vi "shag_start — 6.vi"() -> ()   [LabVIEW 2016]
uses:
  <vilib>/Instr/_visa.llb/VISA Configure Serial Port (Instr).vi
panel:
  out "file":i32
  out "положение в мин 1":i32
  in  "all":T1(tab)
  out "положение шд":i32(knob) scale=-10.0..190.0
  out "текущее положение":string
  out "положение в минутах 1":string
  in  "Минуты":i32 min=-600 max=11400
  in  "Stop двигатель":bool
  in  "Вращение по градусам +":bool
  in  "Вращение по градусам -":bool
  in  "Вернуться в нулевое положение":bool
  in  "Задать текущее положение нулевым":bool
  in  "Установка минут":bool
  in  "Блокировать зеркало №1":bool
  in  "stop":bool
  in  "Выберете COM порт":refnum<visa-resource-name>="COM1"
  in  "Скорость обмена данными":u32(ring)=19200 items=["9600"=9600, "19200"=19200, "38400"=38400, "57600"=57600]
  in  "Число бит на символ":u16=8 min=5 max=8 step=1
  in  "Контроль чётности":enum16{"None", "Odd", "Even", "Mark", "Space"}(ring)
  in  "Стоповый бит":u16(ring)=10 items=["1.0"=10, "1.5"=15, "2.0"=20]
  in  "Контроль переполнения":u16(ring) items=["None"=0, "XON/XOFF"=1, "RTS/CTS"=2, "DTR/DSR"=4]
  # "1 - адресс 1 двигателя\n2 - адресс 2 двигателя\n$0MV\\01+   - запуск всех двигателей в положительном направлении \n$0MS\\00   - остановка всех двигателей\n$0MJ\\04+\\00\\00\\01   - 1 шаг всех двигателей\n$0SS\\01\\10   - скорость 10 для всех двигателей"
  # "Зеркало №1"
  # "Положение:"
  # "Ренгеновская трубка №2:"
  # "Положение ренгеновской трубк:"
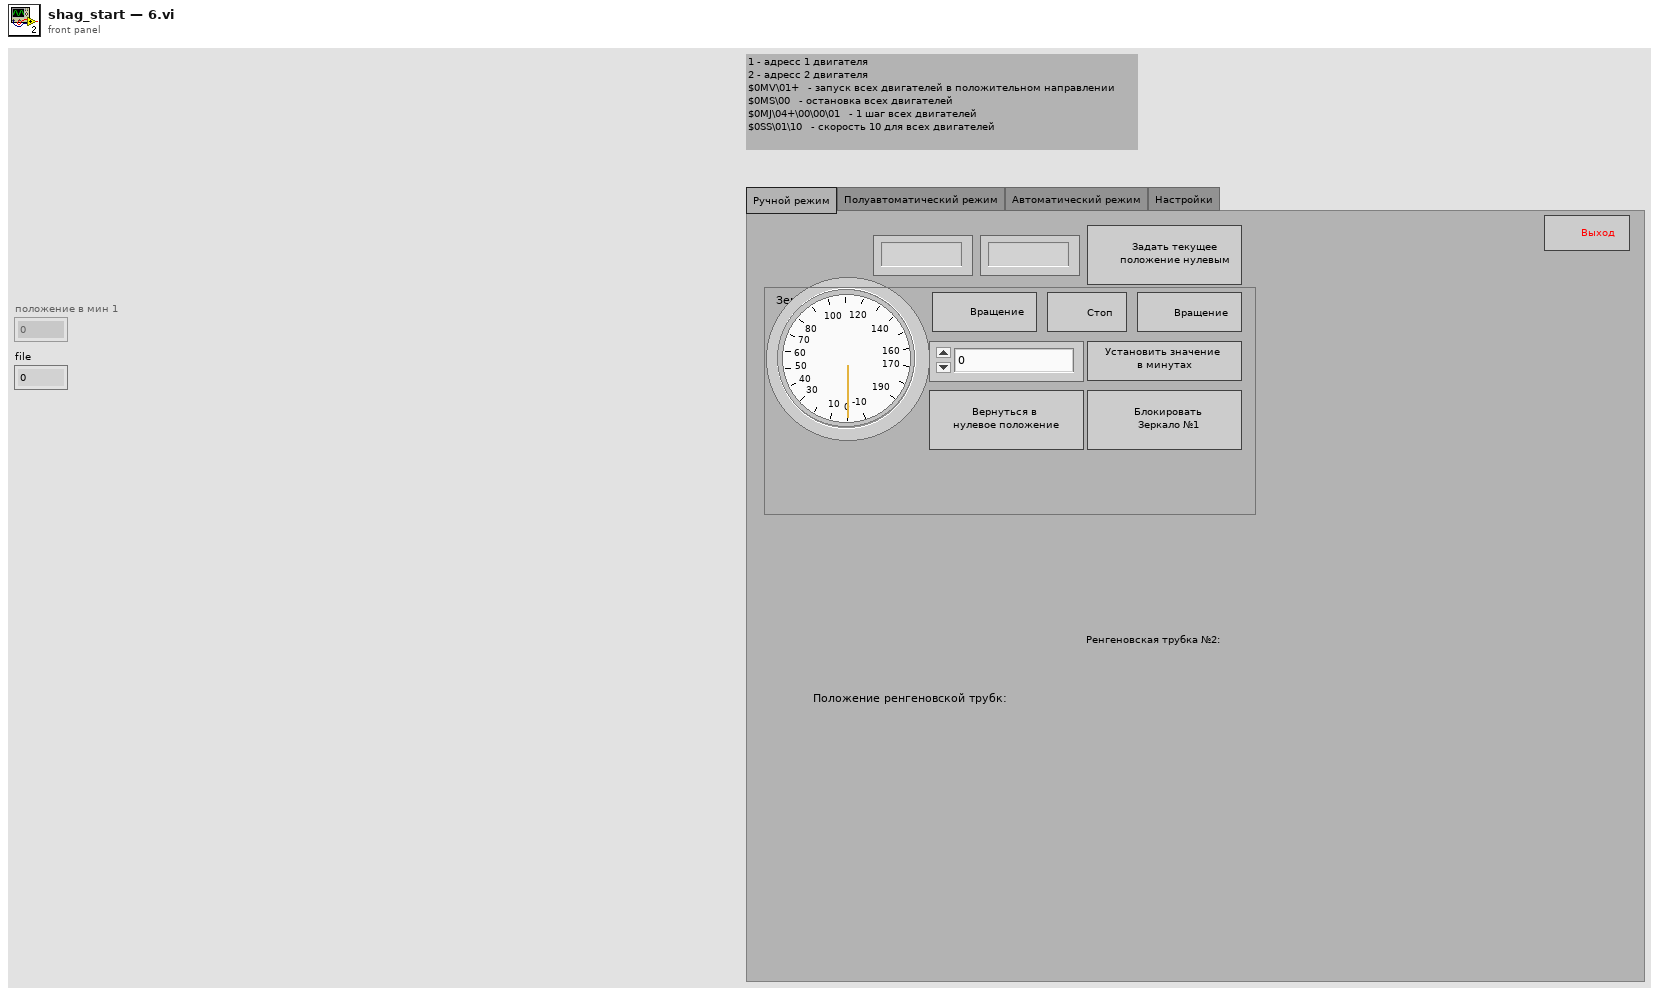
[diagram p1: front panel]
types:
  T1 = enum32{"Ручной режим", "Полуавтоматический режим", "Автоматический режим", "Настройки"}
  T2 = enum16{"open", "replace", "create", "open or create", "replace or create", "replace or create with confirmation"}
  T3 = enum8{"Enabled", "Disabled", "Disabled and Grayed Out"}
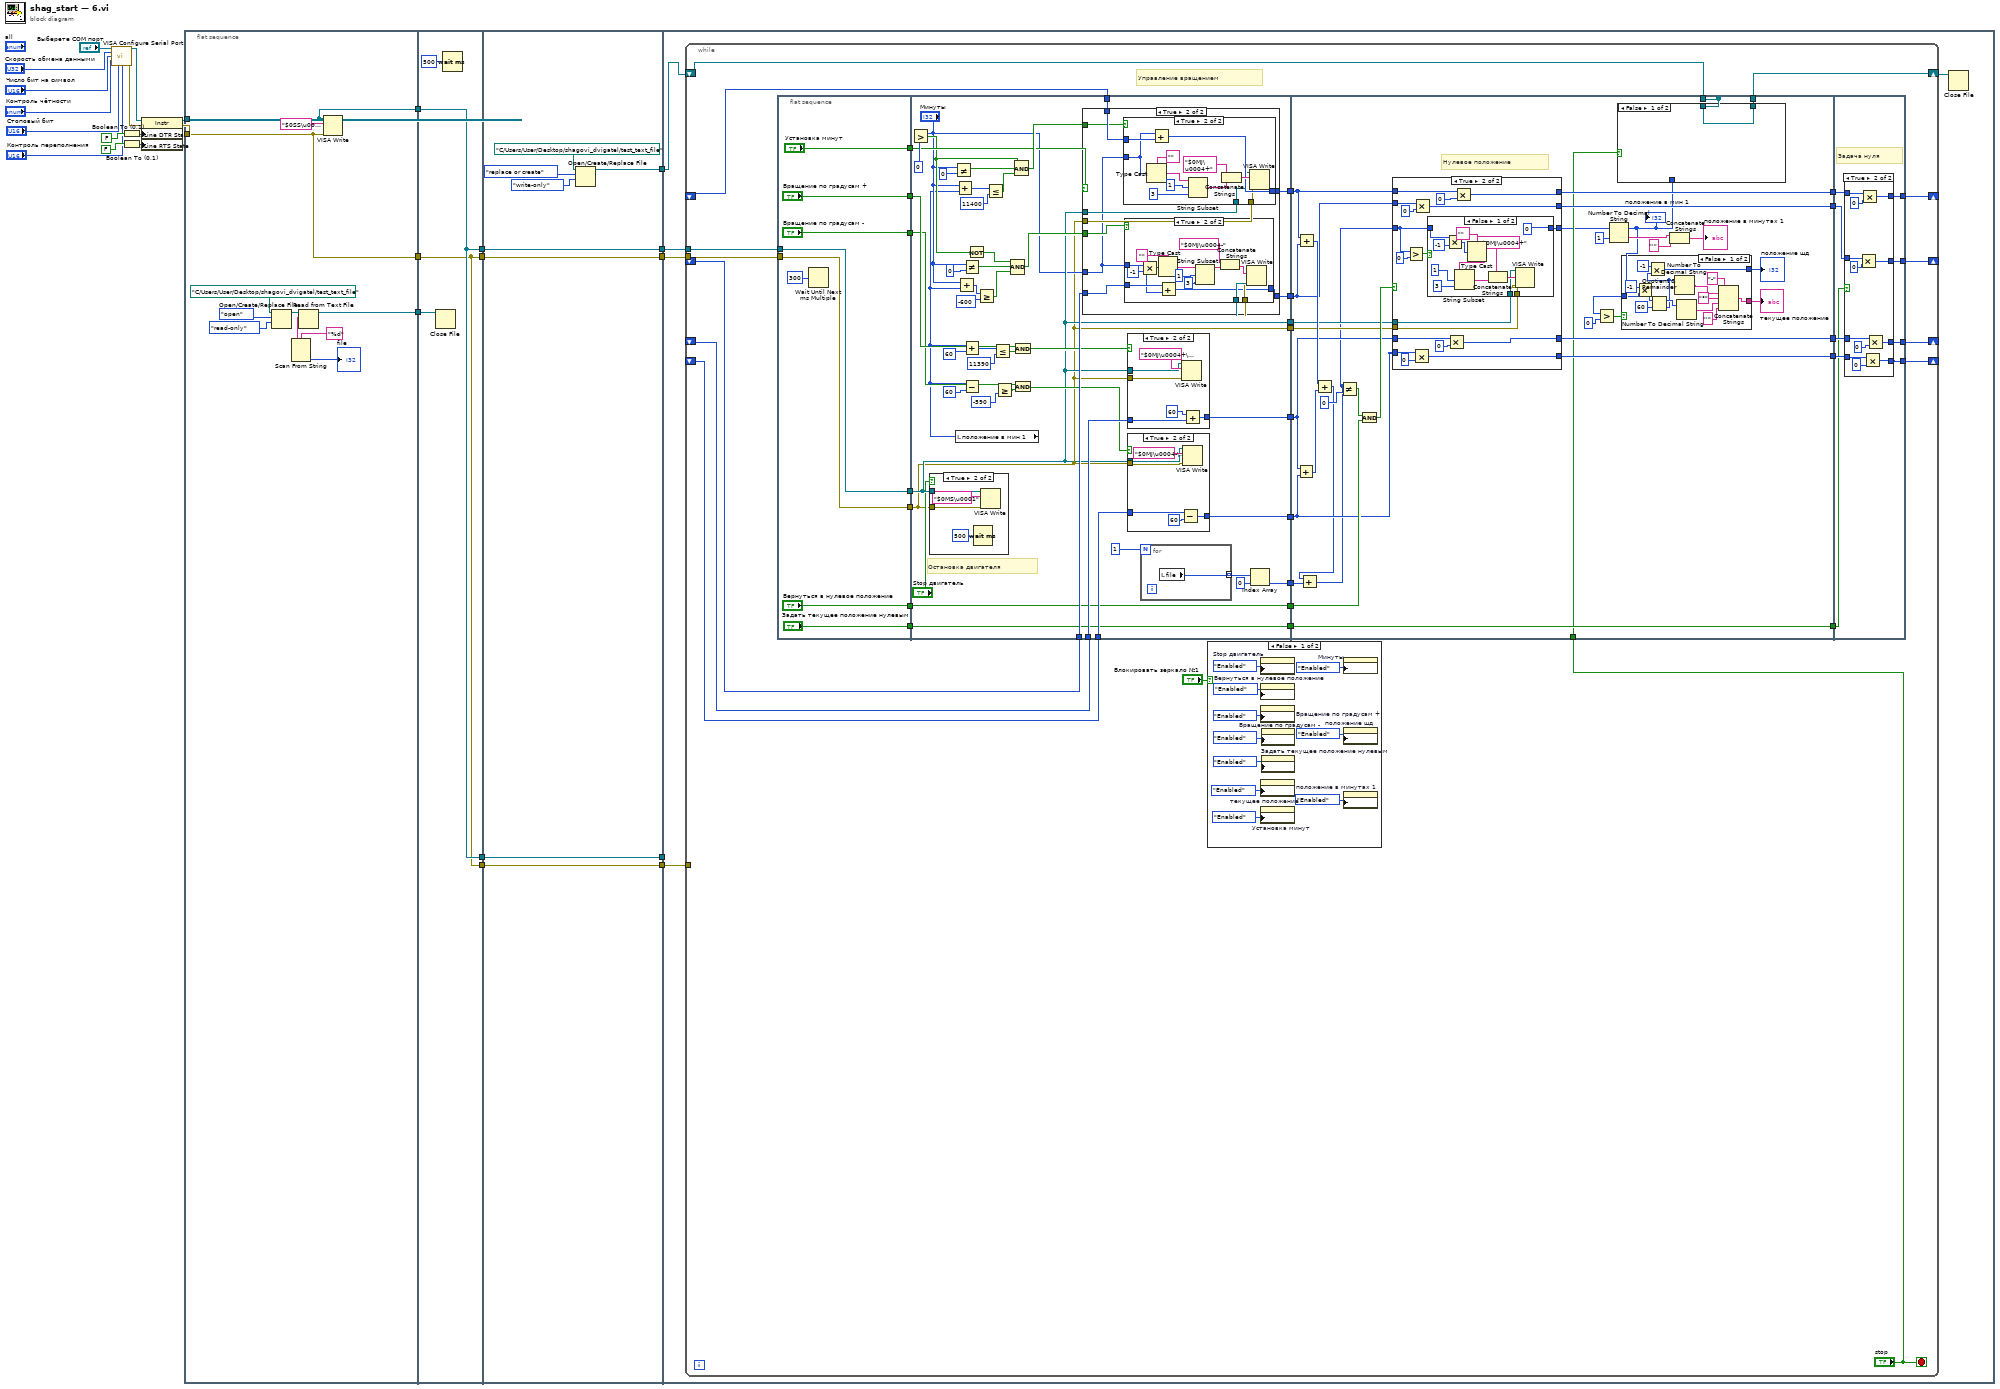
[diagram p0: block diagram]
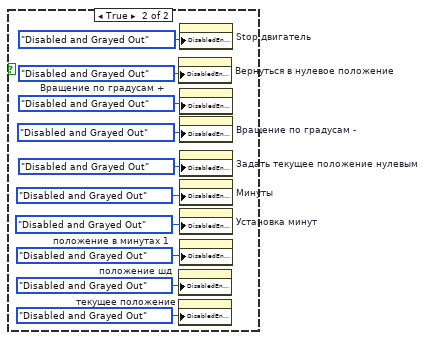
[diagram p2: hidden frame]
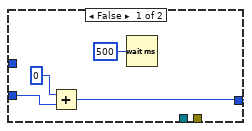
[diagram p4: hidden frame]
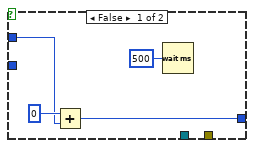
[diagram p5: hidden frame]
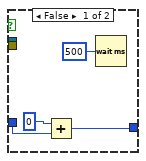
[diagram p7: hidden frame]
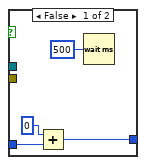
[diagram p8: hidden frame]
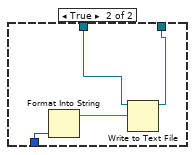
[diagram p9: hidden frame]
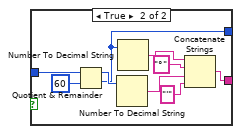
[diagram p10: hidden frame]
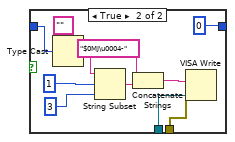
[diagram p12: hidden frame]
diagram:
  n1 = call-poly "VISA Configure Serial Port"("VISA resource name"="Выберете COM порт", "baud rate (9600)"="Скорость обмена данными", "data bits (8)"="Число бит на символ", "parity (0:none)"="Контроль чётности", "stop bits (10: 1 bit)"="Стоповый бит", "flow control (0:none)"="Контроль переполнения") -> ("VISA resource name out"=w24:refnum<visa-resource-name>, "error out"=w23:errorcluster)  [unwired: 8 in]
  n2 = Boolean To (0,1)(Boolean=FALSE ("DTR Write")) -> (0, 1=w25:i16)
  n3 = Boolean To (0,1)(Boolean=FALSE ("DTR Write")) -> (0, 1=w26:i16)
  n4 = property class="Instr"(reference=w24, error in=w23, "Serial Settings:Modem Line Settings:Line DTR State"=w25, "Serial Settings:Modem Line Settings:Line RTS State"=w26) -> (reference out=w22:refnum<visa-resource-name>, error out=w21:errorcluster)
  n5 = flat-sequence {
    tunnel: w22 -> [w36]
    tunnel: w21 -> [w35]
    tunnel: [w36] -> w20
    tunnel: [w35] -> w19
    tunnel: [w29] -> w10
    tunnel: [w40] -> w9
    tunnel: w20 -> [w40]
    tunnel: w19 -> [w39]
    tunnel: [w39] -> w7
    tunnel: [w40] -> w5
    tunnel: [w39] -> w3
    tunnel: w10 -> [w38]
    tunnel: w9 -> [w49]
    tunnel: [w49] -> w8
    tunnel: w7 -> [w48]
    tunnel: [w48] -> w6
    tunnel: w5 -> [w47]
    tunnel: [w47] -> w4
    tunnel: w3 -> [w46]
    tunnel: [w46] -> w2
    tunnel: [w42] -> w1
    tunnel: w8 -> [w54]
    tunnel: w6 -> [w53]
    tunnel: w4 -> [_]
    tunnel: w2 -> [w52]
    tunnel: w1 -> [w51]
    frame #0 {
      n6 = Open/Create/Replace File(file path (use dialog)=path "C:/Users/User/Desktop/shagovi_dvigatel/test_text_file", operation (0:open)=T2."open", access (0:read/write)=enum16{"read/write", "read-only", "write-only"}."read-only") -> (refnum out=w28:refnum<file>)  [unwired: 3 in, 2 out]
      n7 = Read from Text File(file (use dialog)=w28) -> (refnum out=w29:refnum<file>, text=w32:string)  [unwired: 3 in, 2 out]
      n8 = Scan From String(format string="%d", input string=w32) -> (output 1=→"file":i32)  [unwired: 3 in, 3 out]
      n9 = VISA Write(VISA resource name=w36, write buffer="$0SS\u0001\u0010", error in (no error)=w35) -> ()  [unwired: 3 out]
    }
    frame #1 {
      n10 = Close File(refnum=w38) -> ()  [unwired: 1 in, 2 out]
      n11 = Wait (ms)(milliseconds to wait=u32 500) -> ()  [unwired: 1 out]
    }
    frame #2 {
      n12 = Open/Create/Replace File(file path (use dialog)=path "C:/Users/User/Desktop/shagovi_dvigatel/test_text_file", operation (0:open)=T2."replace or create", access (0:read/write)=enum16{"read/write", "read-only", "write-only"}."write-only") -> (refnum out=w42:refnum<file>)  [unwired: 3 in, 2 out]
    }
    frame #3 {
      n13 = while {
        tunnel: w54 -> [w65]
        tunnel: w53 -> [w64]
        shift-right: [w60] -> _
        shift-left: _ -> [w69]
        shift-right: [w61] -> _
        shift-left: _ -> [w68]
        shift-right: [w62] -> _
        shift-left: _ -> [w67]
        shift-right: [w63] -> _
        shift-left: _ -> [w66]
        tunnel: w52 -> [_]
        shift-right: [w55] -> w50
        shift-left: w51 -> [w56]
        stop <- "stop" stop-if-true
        # "Управление вращением"
        n14 = flat-sequence {
          tunnel: w64 -> [w116]
          tunnel: w65 -> [w117]
          tunnel: [w117] -> w89
          tunnel: [w116] -> w88
          tunnel: ["Вращение по градусам +"] -> w87
          tunnel: ["Вращение по градусам -"] -> w86
          tunnel: ["Вернуться в нулевое положение"] -> w85
          tunnel: ["Задать текущее положение нулевым"] -> w84
          tunnel: ["Установка минут"] -> w83
          tunnel: w89 -> [w141]
          tunnel: w88 -> [w123]
          tunnel: [w164] -> w82
          tunnel: w69 -> [w161]
          tunnel: w68 -> [w163]
          tunnel: [w162] -> w81
          tunnel: w67 -> [w160]
          tunnel: w66 -> [w159]
          tunnel: w87 -> [w145]
          tunnel: w86 -> [w144]
          tunnel: [w158] -> w80
          tunnel: [w157] -> w79
          tunnel: [w142] -> w78
          tunnel: w85 -> [w142]
          tunnel: [w123] -> w77
          tunnel: [w141] -> w76
          tunnel: [w140] -> w75
          tunnel: w84 -> [w140]
          tunnel: w83 -> [w134]
          tunnel: [w121] -> w57
          tunnel: w82 -> [w246]
          tunnel: w81 -> [w247]
          tunnel: [w266] -> w74
          tunnel: [w264] -> w73
          tunnel: w80 -> [w248]
          tunnel: w79 -> [w249]
          tunnel: [w255] -> w72
          tunnel: [w262] -> w71
          tunnel: w78 -> [w258]
          tunnel: w77 -> [w254]
          tunnel: w76 -> [w253]
          tunnel: w75 -> [w251]
          tunnel: [w251] -> w70
          tunnel: [w240] -> _
          tunnel: "stop" -> [w243]
          tunnel: w56 -> [w240]
          tunnel: w57 -> [w238]
          tunnel: [w235] -> w55
          tunnel: [w350] -> w60
          tunnel: [w347] -> w61
          tunnel: w74 -> [w349]
          tunnel: w73 -> [w348]
          tunnel: [w346] -> w62
          tunnel: [w345] -> w63
          tunnel: w72 -> [w344]
          tunnel: w71 -> [w343]
          tunnel: w70 -> [w342]
          frame #0 {
            n15 = Wait Until Next ms Multiple(millisecond multiple=u32 300) -> ()  [unwired: 1 out]
          }
          frame #1 {
            # "Остановка двигателя"
            n16 = Greater?(x="Минуты", y=0) -> (0:w132:bool)
            n17 = case shown="True" "Stop двигатель" {
              tunnel: w141 -> [_ w212]
              tunnel: w123 -> [_ w211]
              frame False {
              }
              frame True {
                n18 = Wait (ms)(milliseconds to wait=u32 500) -> ()  [unwired: 1 out]
                n19 = VISA Write(VISA resource name=w212, write buffer="$0MS\u0001", error in (no error)=w211) -> ()  [unwired: 3 out]
              }
            }
            n20 = Not Equal?(x="Минуты", y=0) -> (x != y?=w131:bool)
            n21 = local read "положение в мин 1"() -> (w122:i32)
            n22 = Add(x="Минуты", y=w122) -> (x+y=w155:i32)
            n23 = Add(x="Минуты", y=w122) -> (x+y=w126:i32)
            n24 = Not Equal?(x="Минуты", y=0) -> (x != y?=w129:bool)
            n25 = Add(x=w122, y=60) -> (x+y=w150:i32)
            n26 = Subtract(x=w122, y=60) -> (x-y=w137:i32)
            n27 = Not(x=w132) -> (.not. x?=w133:bool)
            n28 = Greater Or Equal?(x=w126, y=-600) -> (x >= y?=w127:bool)
            n29 = Less Or Equal?(x=w155, y=11400) -> (x <= y?=w130:bool)
            n30 = Less Or Equal?(x=w150, y=11390) -> (x <= y?=w147:bool)
            n31 = Greater Or Equal?(x=w137, y=-590) -> (x >= y?=w138:bool)
            n32 = Compound Arithmetic op=AND(w133, w129, w127) -> (w151:bool)
            n33 = And(x=w145, y=w147) -> (x .and. y?=w146:bool)
            n34 = And(x=w144, y=w138) -> (x .and. y?=w143:bool)
            n35 = Compound Arithmetic op=AND(w132, w131, w130) -> (w153:bool)
            n36 = case shown="True" w134 {
              tunnel: [w167 w176] -> w164
              tunnel: w163 -> [w166 w175]
              tunnel: [w166 w174] -> w162
              tunnel: w161 -> [w167 w173]
              tunnel: w153 -> [_ w172]
              tunnel: w151 -> [_ w171]
              tunnel: w123 -> [_ w170]
              tunnel: w141 -> [_ w169]
              tunnel: "Минуты" -> [_ w168]
              frame False {
              }
              frame True {
                n37 = case shown="True" w172 {
                  tunnel: [w197 w203] -> w176
                  tunnel: w173 -> [w196 w202]
                  tunnel: w170 -> [_ w201]
                  tunnel: w169 -> [_ w200]
                  tunnel: w168 -> [_ w199]
                  frame False {
                    n38 = Add(x=0, y=w196) -> (x+y=w197:i32)
                    n39 = Wait (ms)(milliseconds to wait=u32 500) -> ()  [unwired: 1 out]
                  }
                  frame True {
                    n40 = Type Cast(type="", x=w199) -> (*(type *) &x=w206:string)
                    n41 = Add(x=w199, y=w202) -> (x+y=w203:i32)
                    n42 = String Subset(string=w206, offset (0)=1, length (rest)=3 ("length (rest)")) -> (substring=w205:string)
                    n43 = Concatenate Strings("$0MJ\u0004+" ("write buffer"), w205) -> (w209:string)
                    n44 = VISA Write(VISA resource name=w200, write buffer=w209, error in (no error)=w201) -> ()  [unwired: 3 out]
                  }
                }
                n45 = case shown="True" w171 {
                  tunnel: [w179 w185] -> w174
                  tunnel: w175 -> [w178 w184]
                  tunnel: w169 -> [_ w187]
                  tunnel: w170 -> [_ w186]
                  tunnel: w168 -> [_ w181]
                  frame False {
                    n46 = Add(x=0, y=w178) -> (x+y=w179:i32)
                    n47 = Wait (ms)(milliseconds to wait=u32 500) -> ()  [unwired: 1 out]
                  }
                  frame True {
                    n48 = Multiply(x=w181, y=-1) -> (x*y=w183:i32)
                    n49 = Type Cast(type="", x=w183) -> (*(type *) &x=w190:string)
                    n50 = Add(x=w184, y=w181) -> (x+y=w185:i32)
                    n51 = String Subset(string=w190, offset (0)=1, length (rest)=3 ("length (rest)")) -> (substring=w189:string)
                    n52 = Concatenate Strings("$0MJ\u0004-" ("write buffer"), w189) -> (w193:string)
                    n53 = VISA Write(VISA resource name=w187, write buffer=w193, error in (no error)=w186) -> ()  [unwired: 3 out]
                  }
                }
              }
            }
            n54 = case shown="True" w146 {
              tunnel: [w227 w234] -> w158
              tunnel: w160 -> [w226 w229]
              tunnel: w141 -> [_ w230]
              tunnel: w123 -> [_ w231]
              frame False {
                n55 = Add(x=0, y=w226) -> (x+y=w227:i32)
                n56 = Wait (ms)(milliseconds to wait=u32 500) -> ()  [unwired: 1 out]
              }
              frame True {
                n57 = VISA Write(VISA resource name=w230, write buffer="$0MJ\u0004+\u0000\u0000<", error in (no error)=w231) -> ()  [unwired: 3 out]
                n58 = Add(x=60, y=w229) -> (x+y=w234:i32)
              }
            }
            n59 = case shown="True" w143 {
              tunnel: [w217 w220] -> w157
              tunnel: w159 -> [w216 w219]
              tunnel: w141 -> [_ w223]
              tunnel: w123 -> [_ w222]
              frame False {
                n60 = Add(x=0, y=w216) -> (x+y=w217:i32)
                n61 = Wait (ms)(milliseconds to wait=u32 500) -> ()  [unwired: 1 out]
              }
              frame True {
                n62 = Subtract(x=w219, y=60 ("x")) -> (x-y=w220:i32)
                n63 = VISA Write(VISA resource name=w223, write buffer="$0MJ\u0004-\u0000\u0000<", error in (no error)=w222) -> ()  [unwired: 3 out]
              }
            }
            n64 = for {
              N: 1 -> [_]
              tunnel: [w165] -> w119 mode=indexing
              n65 = local read "file"() -> (w165:i32)
            }
            n66 = Index Array(array=w119, index=0) -> (element=w121:i32)
          }
          frame #2 {
            # "Нулевое положение"
            n67 = Add(x=w248, y=w249) -> (x+y=w259:i32)
            n68 = Add(x=w246, y=w247) -> (x+y=w263:i32)
            n69 = Add(x=w263, y=w259) -> (x+y=w237:i32)
            n70 = Add(x=w237, y=w238) -> (x+y=w236:i32)
            n71 = Not Equal?(x=w236, y=0 ("x")) -> (x != y?=w256:bool)
            n72 = And(x=w256, y=w258) -> (x .and. y?=w265:bool)
            n73 = case shown="True" w265 {
              tunnel: [w295 w317] -> w239
              tunnel: w246 -> [w299 w314]
              tunnel: [w299 w313] -> w266
              tunnel: [w298 w312] -> w264
              tunnel: w236 -> [w295 w306]
              tunnel: [w296 w308] -> w262
              tunnel: [w297 w305] -> w255
              tunnel: w247 -> [w298 w304]
              tunnel: w254 -> [_ w303]
              tunnel: w253 -> [_ w302]
              tunnel: w248 -> [w297 w301]
              tunnel: w249 -> [w296 w300]
              frame False {
              }
              frame True {
                n74 = Greater?(x=w306, y=0) -> (0:w307:bool)
                n75 = Multiply(x=w300, y=0) -> (x*y=w308:i32)
                n76 = Multiply(x=w304, y=0) -> (x*y=w312:i32)
                n77 = case shown="False" w307 {
                  tunnel: w306 -> [w322 w335]
                  tunnel: [0 0] -> w317
                  tunnel: w302 -> [w319 w332]
                  tunnel: w303 -> [w318 w331]
                  frame False {
                    n78 = Multiply(x=w322, y=-1) -> (x*y=w320:i32)
                    n79 = Type Cast(type="", x=w320) -> (*(type *) &x=w326:string)
                    n80 = String Subset(string=w326, offset (0)=1, length (rest)=3 ("length (rest)")) -> (substring=w325:string)
                    n81 = Concatenate Strings("$0MJ\u0004+" ("write buffer"), w325) -> (w329:string)
                    n82 = VISA Write(VISA resource name=w319, write buffer=w329, error in (no error)=w318) -> ()  [unwired: 3 out]
                  }
                  frame True {
                    n83 = Type Cast(type="", x=w335) -> (*(type *) &x=w338:string)
                    n84 = String Subset(string=w338, offset (0)=1, length (rest)=3 ("length (rest)")) -> (substring=w337:string)
                    n85 = Concatenate Strings("$0MJ\u0004-" ("write buffer"), w337) -> (w333:string)
                    n86 = VISA Write(VISA resource name=w332, write buffer=w333, error in (no error)=w331) -> ()  [unwired: 3 out]
                  }
                }
                n87 = Multiply(x=w301, y=0) -> (x*y=w305:i32)
                n88 = Multiply(x=w314, y=0) -> (x*y=w313:i32)
              }
            }
            "положение в мин 1" <- w239
            n89 = Greater?(x=w239, y=0) -> (0:w261:bool)
            n90 = Number To Decimal String(number=w239, width (-)=i16 1) -> (decimal integer string=w242:string)
            n91 = case shown="False" w243 {
              tunnel: w240 -> [w267 w269]
              tunnel: w239 -> [_ w270]
              tunnel: [w267 w268] -> w235
              frame False {
              }
              frame True {
                n92 = Format Into String(w270) -> (resulting string=w271:string)  [unwired: 3 in, 1 out]
                n93 = Write to Text File(file (use dialog)=w269, text=w271) -> (refnum out=w268:refnum<file>)  [unwired: 2 in, 2 out]
              }
            }
            n94 = case shown="False" w261 {
              tunnel: w239 -> [w278 w294]
              tunnel: [w282 w288] -> w252
              tunnel: [w272 w286] -> w250
              frame False {
                n95 = Multiply(x=-1, y=w278) -> (x*y=w277:i32)
                n96 = Quotient & Remainder(x=w277, y=60) -> (x-y*floor(x/y)=w281:i32, floor(x/y)=w273:i32)
                n97 = Multiply(x=-1, y=w273) -> (x*y=w272:i32)
                n98 = Number To Decimal String(number=w273) -> (decimal integer string=w279:string)  [unwired: 1 in]
                n99 = Number To Decimal String(number=w281) -> (decimal integer string=w280:string)  [unwired: 1 in]
                n100 = Concatenate Strings("-" ("string"), w279, "°" ("string"), w280, "'" ("string")) -> (w282:string)
              }
              frame True {
                n101 = Quotient & Remainder(x=w294, y=60) -> (x-y*floor(x/y)=w287:i32, floor(x/y)=w286:i32)
                n102 = Number To Decimal String(number=w287) -> (decimal integer string=w289:string)  [unwired: 1 in]
                n103 = Number To Decimal String(number=w286) -> (decimal integer string=w290:string)  [unwired: 1 in]
                n104 = Concatenate Strings(w290, "°" ("string"), w289, "'" ("string")) -> (w288:string)
              }
            }
            "положение шд" <- w250
            "текущее положение" <- w252
            n105 = Concatenate Strings(w242, "'" ("string")) -> (→"положение в минутах 1":string)
          }
          frame #3 {
            # "Задача нуля"
            n106 = case shown="True" w342 {
              tunnel: [w354 w365] -> w350
              tunnel: w349 -> [w354 w366]
              tunnel: w348 -> [w353 w362]
              tunnel: [w353 w361] -> w347
              tunnel: [w352 w358] -> w346
              tunnel: [w351 w357] -> w345
              tunnel: w344 -> [w352 w356]
              tunnel: w343 -> [w351 w355]
              frame False {
              }
              frame True {
                n107 = Multiply(x=w362, y=0) -> (x*y=w361:i32)
                n108 = Multiply(x=w366, y=0) -> (x*y=w365:i32)
                n109 = Multiply(x=w355, y=0) -> (x*y=w357:i32)
                n110 = Multiply(x=w356, y=0) -> (x*y=w358:i32)
              }
            }
          }
        }
        n111 = case shown="False" "Блокировать зеркало №1" {
          frame False {
            n112 = property on="Stop двигатель" class="Bool"("DisabledEnum"=T3."Enabled" ("Disabled")) -> ()  [unwired: 2 in, 2 out]
            n113 = property on="Вернуться в нулевое положение" class="Bool"("DisabledEnum"=T3."Enabled" ("Disabled")) -> ()  [unwired: 2 in, 2 out]
            n114 = property on="Вращение по градусам +" class="Bool"("DisabledEnum"=T3."Enabled" ("Disabled")) -> ()  [unwired: 2 in, 2 out]
            n115 = property on="текущее положение" class="Str"("DisabledEnum"=T3."Enabled" ("Disabled")) -> ()  [unwired: 2 in, 2 out]
            n116 = property on="Установка минут" class="Bool"("DisabledEnum"=T3."Enabled" ("Disabled")) -> ()  [unwired: 2 in, 2 out]
            n117 = property on="Вращение по градусам -" class="Bool"("DisabledEnum"=T3."Enabled" ("Disabled")) -> ()  [unwired: 2 in, 2 out]
            n118 = property on="Задать текущее положение нулевым" class="Bool"("DisabledEnum"=T3."Enabled" ("Disabled")) -> ()  [unwired: 2 in, 2 out]
            n119 = property on="Минуты" class="DigNum (strict)"("DisabledEnum"=T3."Enabled" ("Disabled")) -> ()  [unwired: 2 in, 2 out]
            n120 = property on="положение шд" class="Knob (strict)"("DisabledEnum"=T3."Enabled" ("Disabled")) -> ()  [unwired: 2 in, 2 out]
            n121 = property on="положение в минутах 1" class="Str"("DisabledEnum"=T3."Enabled" ("Disabled")) -> ()  [unwired: 2 in, 2 out]
          }
          frame True {
            n122 = property on="Вернуться в нулевое положение" class="Bool"("DisabledEnum"=T3."Disabled and Grayed Out" ("Disabled")) -> ()  [unwired: 2 in, 2 out]
            n123 = property on="положение шд" class="Knob (strict)"("DisabledEnum"=T3."Disabled and Grayed Out" ("Disabled")) -> ()  [unwired: 2 in, 2 out]
            n124 = property on="текущее положение" class="Str"("DisabledEnum"=T3."Disabled and Grayed Out" ("Disabled")) -> ()  [unwired: 2 in, 2 out]
            n125 = property on="Stop двигатель" class="Bool"("DisabledEnum"=T3."Disabled and Grayed Out" ("Disabled")) -> ()  [unwired: 2 in, 2 out]
            n126 = property on="Вращение по градусам +" class="Bool"("DisabledEnum"=T3."Disabled and Grayed Out" ("Disabled")) -> ()  [unwired: 2 in, 2 out]
            n127 = property on="Вращение по градусам -" class="Bool"("DisabledEnum"=T3."Disabled and Grayed Out" ("Disabled")) -> ()  [unwired: 2 in, 2 out]
            n128 = property on="Задать текущее положение нулевым" class="Bool"("DisabledEnum"=T3."Disabled and Grayed Out" ("Disabled")) -> ()  [unwired: 2 in, 2 out]
            n129 = property on="Минуты" class="DigNum (strict)"("DisabledEnum"=T3."Disabled and Grayed Out" ("Disabled")) -> ()  [unwired: 2 in, 2 out]
            n130 = property on="Установка минут" class="Bool"("DisabledEnum"=T3."Disabled and Grayed Out" ("Disabled")) -> ()  [unwired: 2 in, 2 out]
            n131 = property on="положение в минутах 1" class="Str"("DisabledEnum"=T3."Disabled and Grayed Out" ("Disabled")) -> ()  [unwired: 2 in, 2 out]
          }
        }
      }
      n132 = Close File(refnum=w50) -> ()  [unwired: 1 in, 2 out]
    }
  }
